vi "ByteArrayToBitArray.vi"(3 "Flip Endian":bool=TRUE, 6 "Byte Array In":u8[](array[numeric])) -> (1 "Bit Array Out":bool[](array[boolean]))   [LabVIEW 2014]
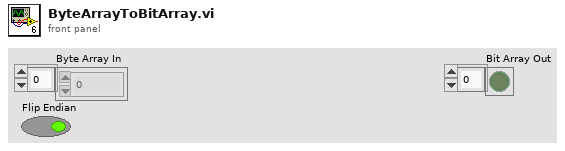
[diagram p1: front panel]
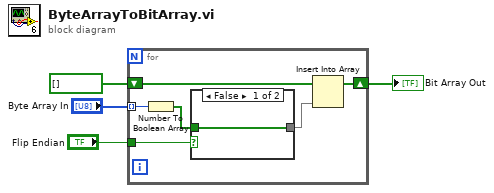
[diagram p0: block diagram]
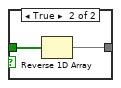
[diagram p2: hidden frame]
diagram:
  n1 = for {
    shift-right: [w9] -> w2
    shift-left: bool[] [] -> [w10]
    tunnel: "Byte Array In" -> [w8] mode=indexing
    tunnel: "Flip Endian" -> [w7]
    n2 = Number To Boolean Array(number=w8) -> (Boolean array=w6:bool[])
    n3 = case shown="False" w7 {
      tunnel: w6 -> [w11 w13]
      tunnel: [w11 w12] -> w5
      frame False {
      }
      frame True {
        n4 = Reverse 1D Array(array=w13) -> (reversed array=w12:bool[])
      }
    }
    n5 = Insert Into Array(array=w10, new element=w5) -> (w9:bool[])  [unwired: 1 in]
  }
  "Bit Array Out" <- w2
